vi "Tester.vi"() -> ()   [LabVIEW 2019, in "BigMAQ.lvclass"]
uses:
  BigMAQ.lvclass
  <userlib>/Levylab/Relay Box/Typedefs/Resistor--enum.ctl
  BigMAQ.lvclass/BigMAQ.ctl
  <userlib>/Levylab/Relay Box/Relay-Box.lvclass
panel:
  out "Array":i32[](array[numeric])
  out "x = y?":bool
  out "Image":T1(plugin-control)
  in  "Collapse":bool
  out "Render":T1(plugin-control)
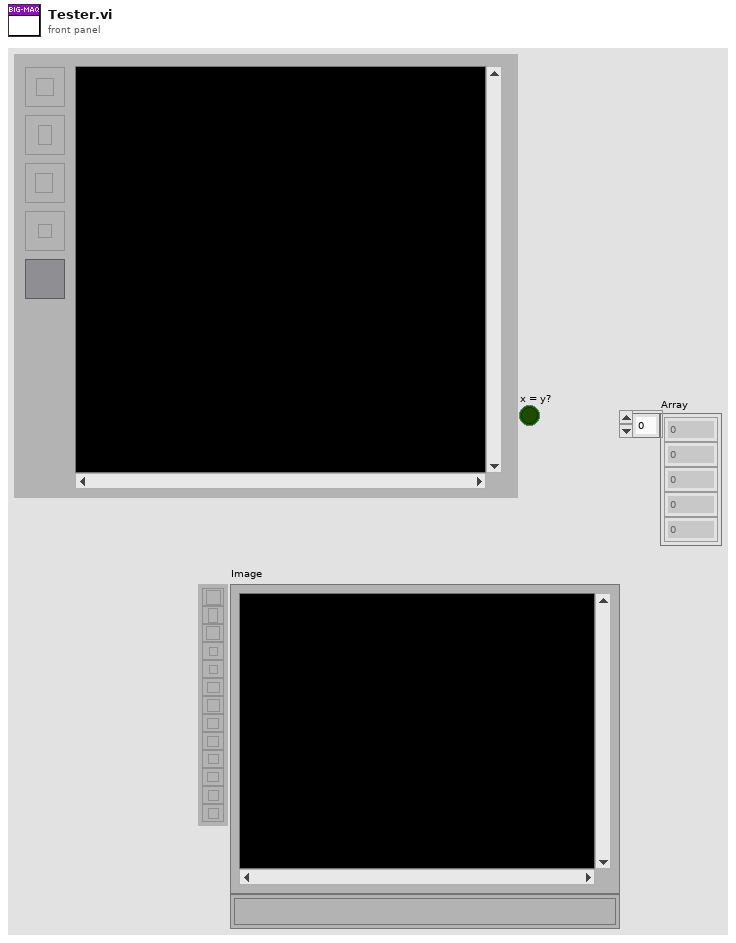
[diagram p1: front panel]
types:
  T1 = typedef "IMAQ Image.ctl" = refnum<image>
  T2 = typedef "Relay-Box.lvclass/Resistor--enum.ctl" = enum16{"open", "discharge tip", "0 ohms", "100k ohm", "10M ohm", "1G ohm"}
  T3 = cluster{"Name":string, "Litho":cluster{"X":dbl, "Y":dbl, "Speed":dbl, "Voltage":dbl}[], "Set Resistance":T2, "Meta":variant}[]
  T4 = cluster{"Name":string, "Litho":cluster{"X":dbl, "Y":dbl, "Speed":dbl, "Voltage":dbl}[], "Set Resistance":T2, "Meta":variant}
  T5 = cluster{"X":dbl, "Y":dbl, "Speed":dbl, "Voltage":dbl}[]
  T6 = cluster{"X":dbl, "Y":dbl, "Speed":dbl, "Voltage":dbl}
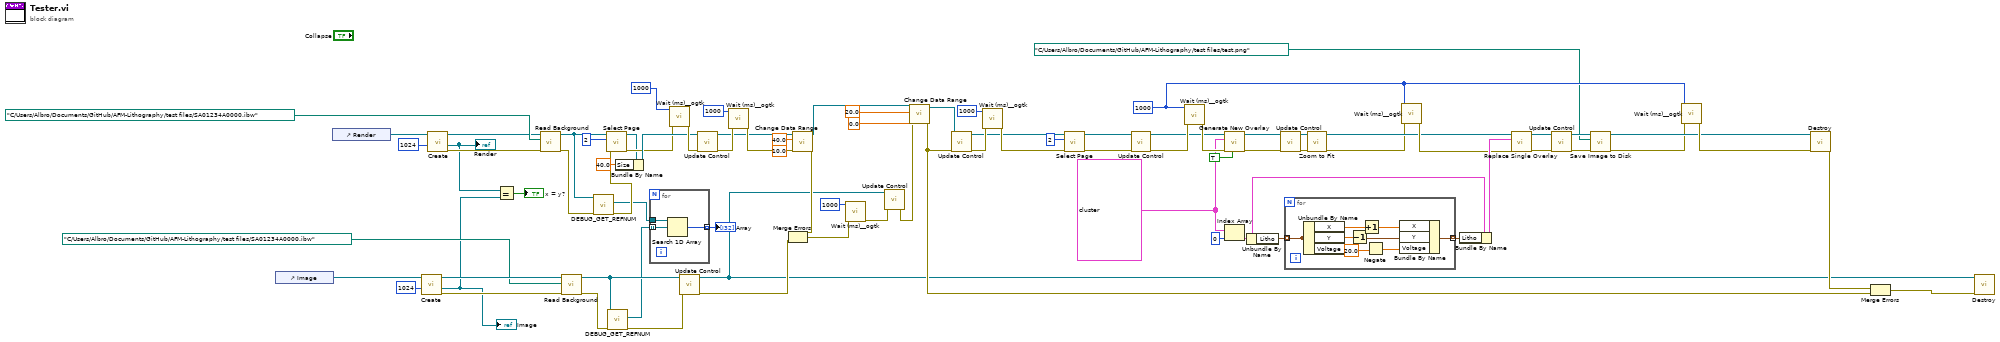
[diagram p0: block diagram]
diagram:
  w63 = T3 [{"Name"="p0", "Litho"=array[26726 elements], "Set Resistance"=enum."1G ohm", "Meta"=variant}, {"Name"="p1", "Litho"=array[12429 elements], "Set Resistance"=enum."1G ohm", "Meta"=variant}, {"Name"="p2", "Litho"=array[8953 elements], "Set Resistance"=enum."1G ohm", "Meta"=variant}, {"Name"="p3", "Litho"=array[11526 elements], "Set Resistance"=enum."1G ohm", "Meta"=variant}, {"Name"="p4", "Litho"=array[11508 elements], "Set Resistance"=enum."1G ohm", "Meta"=variant}, {"Name"="p5", "Litho"=array[11203 elements], "Set Resistance"=enum."1G ohm", "Meta"=variant}, {"Name"="p6", "Litho"=array[9937 elements], "Set Resistance"=enum."1G ohm", "Meta"=variant}, {"Name"="p7", "Litho"=array[9921 elements], "Set Resistance"=enum."1G ohm", "Meta"=variant}, {"Name"="p8", "Litho"=array[9914 elements], "Set Resistance"=enum."1G ohm", "Meta"=variant}, {"Name"="p9", "Litho"=array[57227 elements], "Set Resistance"=enum."1G ohm", "Meta"=variant}, {"Name"="f0", "Litho"=[{"X"=5.710942899999999, "Y"=17.975706, "Speed"=10.0, "Voltage"=10.0}, {"X"=6.38914543287037, "Y"=17.336981402777777, "Speed"=10.0, "Voltage"=10.0}, {"X"=7.122646896296295, "Y"=16.828463888888884, "Speed"=10.0, "Voltage"=10.0}, {"X"=7.9028574875, "Y"=16.429927874999997, "Speed"=10.0, "Voltage"=10.0}, {"X"=8.721187403703704, "Y"=16.121147777777775, "Speed"=10.0, "Voltage"=10.0}, {"X"=9.56904684212963, "Y"=15.88189801388889, "Speed"=10.0, "Voltage"=10.0}, {"X"=10.437846, "Y"=15.691952999999998, "Speed"=10.0, "Voltage"=10.0}, {"X"=9.579383034722223, "Y"=15.781785605555555, "Speed"=10.0, "Voltage"=10.0}, {"X"=8.740301544444446, "Y"=15.905736977777776, "Speed"=10.0, "Voltage"=10.0}, {"X"=7.9277050875, "Y"=16.079518349999997, "Speed"=10.0, "Voltage"=10.0}, {"X"=7.148697222222221, "Y"=16.31884095555555, "Speed"=10.0, "Voltage"=10.0}, {"X"=6.410381506944445, "Y"=16.639416027777777, "Speed"=10.0, "Voltage"=10.0}, {"X"=5.719861499999999, "Y"=17.056954799999996, "Speed"=10.0, "Voltage"=10.0}, {"X"=5.728780099999999, "Y"=16.138203599999997, "Speed"=10.0, "Voltage"=10.0}, {"X"=6.431617581018519, "Y"=15.941850652777777, "Speed"=10.0, "Voltage"=10.0}, {"X"=7.174747548148147, "Y"=15.809218022222218, "Speed"=10.0, "Voltage"=10.0}, {"X"=7.952552687499999, "Y"=15.729108824999997, "Speed"=10.0, "Voltage"=10.0}, {"X"=8.759415685185186, "Y"=15.690326177777777, "Speed"=10.0, "Voltage"=10.0}, {"X"=9.589719227314816, "Y"=15.68167319722222, "Speed"=10.0, "Voltage"=10.0}, {"X"=10.437846, "Y"=15.691952999999998, "Speed"=10.0, "Voltage"=10.0}, {"X"=9.60005541990741, "Y"=15.581560788888888, "Speed"=10.0, "Voltage"=10.0}, {"X"=8.778529825925926, "Y"=15.474915377777776, "Speed"=10.0, "Voltage"=10.0}, {"X"=7.9774002875, "Y"=15.378699299999997, "Speed"=10.0, "Voltage"=10.0}, {"X"=7.200797874074075, "Y"=15.299595088888886, "Speed"=10.0, "Voltage"=10.0}, {"X"=6.452853655092593, "Y"=15.244285277777777, "Speed"=10.0, "Voltage"=10.0}, {"X"=5.737698699999999, "Y"=15.219452399999996, "Speed"=10.0, "Voltage"=10.0}, {"X"=5.7466173, "Y"=14.300701199999995, "Speed"=10.0, "Voltage"=10.0}, {"X"=6.474089729166667, "Y"=14.546719902777777, "Speed"=10.0, "Voltage"=10.0}, {"X"=7.226848200000001, "Y"=14.789972155555553, "Speed"=10.0, "Voltage"=10.0}, {"X"=8.0022478875, "Y"=15.028289774999998, "Speed"=10.0, "Voltage"=10.0}, {"X"=8.797643966666667, "Y"=15.259504577777776, "Speed"=10.0, "Voltage"=10.0}, {"X"=9.610391612500003, "Y"=15.481448380555555, "Speed"=10.0, "Voltage"=10.0}, {"X"=10.437846, "Y"=15.691952999999998, "Speed"=10.0, "Voltage"=10.0}, {"X"=9.620727805092596, "Y"=15.381335972222221, "Speed"=10.0, "Voltage"=10.0}, {"X"=8.816758107407408, "Y"=15.044093777777777, "Speed"=10.0, "Voltage"=10.0}, {"X"=8.027095487499999, "Y"=14.677880249999998, "Speed"=10.0, "Voltage"=10.0}, {"X"=7.252898525925927, "Y"=14.280349222222222, "Speed"=10.0, "Voltage"=10.0}, {"X"=6.495325803240741, "Y"=13.849154527777776, "Speed"=10.0, "Voltage"=10.0}, {"X"=5.7555359, "Y"=13.381949999999996, "Speed"=10.0, "Voltage"=10.0}], "Set Resistance"=enum."open", "Meta"=variant}, {"Name"="f1", "Litho"=[{"X"=13.400891999999999, "Y"=10.059383, "Speed"=10.0, "Voltage"=10.0}, {"X"=14.039616597222224, "Y"=10.737586125, "Speed"=10.0, "Voltage"=10.0}, {"X"=14.548134111111112, "Y"=11.471087999999998, "Speed"=10.0, "Voltage"=10.0}, {"X"=14.946670125, "Y"=12.251298874999998, "Speed"=10.0, "Voltage"=10.0}, {"X"=15.255450222222224, "Y"=13.069628999999999, "Speed"=10.0, "Voltage"=10.0}, {"X"=15.494699986111113, "Y"=13.917488625, "Speed"=10.0, "Voltage"=10.0}, {"X"=15.684645, "Y"=14.786287999999999, "Speed"=10.0, "Voltage"=10.0}, {"X"=15.594812394444446, "Y"=13.92782480462963, "Speed"=10.0, "Voltage"=10.0}, {"X"=15.470861022222223, "Y"=13.088743103703703, "Speed"=10.0, "Voltage"=10.0}, {"X"=15.29707965, "Y"=12.276146424999999, "Speed"=10.0, "Voltage"=10.0}, {"X"=15.057757044444447, "Y"=11.497138296296296, "Speed"=10.0, "Voltage"=10.0}, {"X"=14.737181972222224, "Y"=10.758822245370371, "Speed"=10.0, "Voltage"=10.0}, {"X"=14.3196432, "Y"=10.0683018, "Speed"=10.0, "Voltage"=10.0}, {"X"=15.2383944, "Y"=10.0772206, "Speed"=10.0, "Voltage"=10.0}, {"X"=15.434747347222224, "Y"=10.780058365740741, "Speed"=10.0, "Voltage"=10.0}, {"X"=15.56737997777778, "Y"=11.523188592592591, "Speed"=10.0, "Voltage"=10.0}, {"X"=15.647489175, "Y"=12.300993975, "Speed"=10.0, "Voltage"=10.0}, {"X"=15.686271822222224, "Y"=13.107857207407406, "Speed"=10.0, "Voltage"=10.0}, {"X"=15.69492480277778, "Y"=13.938160984259259, "Speed"=10.0, "Voltage"=10.0}, {"X"=15.684645, "Y"=14.786287999999999, "Speed"=10.0, "Voltage"=10.0}, {"X"=15.795037211111115, "Y"=13.94849716388889, "Speed"=10.0, "Voltage"=10.0}, {"X"=15.901682622222225, "Y"=13.12697131111111, "Speed"=10.0, "Voltage"=10.0}, {"X"=15.9978987, "Y"=12.325841525000001, "Speed"=10.0, "Voltage"=10.0}, {"X"=16.077002911111112, "Y"=11.549238888888887, "Speed"=10.0, "Voltage"=10.0}, {"X"=16.132312722222224, "Y"=10.80129448611111, "Speed"=10.0, "Voltage"=10.0}, {"X"=16.1571456, "Y"=10.0861394, "Speed"=10.0, "Voltage"=10.0}, {"X"=17.075896800000002, "Y"=10.0950582, "Speed"=10.0, "Voltage"=10.0}, {"X"=16.829878097222224, "Y"=10.82253060648148, "Speed"=10.0, "Voltage"=10.0}, {"X"=16.586625844444445, "Y"=11.575289185185184, "Speed"=10.0, "Voltage"=10.0}, {"X"=16.348308225, "Y"=12.350689075, "Speed"=10.0, "Voltage"=10.0}, {"X"=16.117093422222226, "Y"=13.146085414814813, "Speed"=10.0, "Voltage"=10.0}, {"X"=15.895149619444448, "Y"=13.958833343518519, "Speed"=10.0, "Voltage"=10.0}, {"X"=15.684645, "Y"=14.786287999999999, "Speed"=10.0, "Voltage"=10.0}, {"X"=15.99526202777778, "Y"=13.969169523148148, "Speed"=10.0, "Voltage"=10.0}, {"X"=16.332504222222223, "Y"=13.165199518518516, "Speed"=10.0, "Voltage"=10.0}, {"X"=16.69871775, "Y"=12.375536625, "Speed"=10.0, "Voltage"=10.0}, {"X"=17.096248777777777, "Y"=11.601339481481482, "Speed"=10.0, "Voltage"=10.0}, {"X"=17.527443472222224, "Y"=10.84376672685185, "Speed"=10.0, "Voltage"=10.0}, {"X"=17.994648, "Y"=10.103976999999999, "Speed"=10.0, "Voltage"=10.0}], "Set Resistance"=enum."open", "Meta"=variant}, {"Name"="f2", "Litho"=[{"X"=18.739549, "Y"=9.9886728, "Speed"=10.0, "Voltage"=10.0}, {"X"=19.378273597222226, "Y"=10.666875587962963, "Speed"=10.0, "Voltage"=10.0}, {"X"=19.88679111111111, "Y"=11.400377237037036, "Speed"=10.0, "Voltage"=10.0}, {"X"=20.285327125000002, "Y"=12.180587974999998, "Speed"=10.0, "Voltage"=10.0}, {"X"=20.59410722222222, "Y"=12.998918029629628, "Speed"=10.0, "Voltage"=10.0}, {"X"=20.833356986111113, "Y"=13.846777628703705, "Speed"=10.0, "Voltage"=10.0}, {"X"=21.023302, "Y"=14.715577, "Speed"=10.0, "Voltage"=10.0}, {"X"=20.933469394444444, "Y"=13.857113821481484, "Speed"=10.0, "Voltage"=10.0}, {"X"=20.80951802222222, "Y"=13.018032171851852, "Speed"=10.0, "Voltage"=10.0}, {"X"=20.63573665, "Y"=12.20543558, "Speed"=10.0, "Voltage"=10.0}, {"X"=20.39641404444444, "Y"=11.426427574814815, "Speed"=10.0, "Voltage"=10.0}, {"X"=20.07583897222223, "Y"=10.688111685185184, "Speed"=10.0, "Voltage"=10.0}, {"X"=19.6583002, "Y"=9.99759144, "Speed"=10.0, "Voltage"=10.0}, {"X"=20.5770514, "Y"=10.00651008, "Speed"=10.0, "Voltage"=10.0}, {"X"=20.77340434722223, "Y"=10.709347782407407, "Speed"=10.0, "Voltage"=10.0}, {"X"=20.906036977777777, "Y"=11.452477912592592, "Speed"=10.0, "Voltage"=10.0}, {"X"=20.986146175, "Y"=12.230283184999998, "Speed"=10.0, "Voltage"=10.0}, {"X"=21.024928822222222, "Y"=13.037146314074073, "Speed"=10.0, "Voltage"=10.0}, {"X"=21.03358180277778, "Y"=13.867450014259262, "Speed"=10.0, "Voltage"=10.0}, {"X"=21.023302, "Y"=14.715577, "Speed"=10.0, "Voltage"=10.0}, {"X"=21.133694211111113, "Y"=13.877786207037037, "Speed"=10.0, "Voltage"=10.0}, {"X"=21.240339622222223, "Y"=13.056260456296295, "Speed"=10.0, "Voltage"=10.0}, {"X"=21.336555699999998, "Y"=12.255130789999999, "Speed"=10.0, "Voltage"=10.0}, {"X"=21.415659911111113, "Y"=11.47852825037037, "Speed"=10.0, "Voltage"=10.0}, {"X"=21.47096972222223, "Y"=10.73058387962963, "Speed"=10.0, "Voltage"=10.0}, {"X"=21.495802599999998, "Y"=10.01542872, "Speed"=10.0, "Voltage"=10.0}, {"X"=22.414553799999997, "Y"=10.024347359999998, "Speed"=10.0, "Voltage"=10.0}, {"X"=22.16853509722223, "Y"=10.751819976851852, "Speed"=10.0, "Voltage"=10.0}, {"X"=21.925282844444446, "Y"=11.50457858814815, "Speed"=10.0, "Voltage"=10.0}, {"X"=21.686965224999998, "Y"=12.279978394999997, "Speed"=10.0, "Voltage"=10.0}, {"X"=21.455750422222224, "Y"=13.075374598518518, "Speed"=10.0, "Voltage"=10.0}, {"X"=21.233806619444444, "Y"=13.888122399814815, "Speed"=10.0, "Voltage"=10.0}, {"X"=21.023302, "Y"=14.715577, "Speed"=10.0, "Voltage"=10.0}, {"X"=21.333919027777778, "Y"=13.898458592592593, "Speed"=10.0, "Voltage"=10.0}, {"X"=21.671161222222224, "Y"=13.09448874074074, "Speed"=10.0, "Voltage"=10.0}, {"X"=22.037374749999998, "Y"=12.304825999999998, "Speed"=10.0, "Voltage"=10.0}, {"X"=22.43490577777778, "Y"=11.530628925925928, "Speed"=10.0, "Voltage"=10.0}, {"X"=22.86610047222223, "Y"=10.773056074074074, "Speed"=10.0, "Voltage"=10.0}, {"X"=23.333305, "Y"=10.033266, "Speed"=10.0, "Voltage"=10.0}], "Set Resistance"=enum."open", "Meta"=variant}, {"Name"="f3", "Litho"=[{"X"=8.1004383, "Y"=10.879120000000002, "Speed"=10.0, "Voltage"=10.0}, {"X"=8.862424111111112, "Y"=11.415129314814816, "Speed"=10.0, "Voltage"=10.0}, {"X"=9.507971822222222, "Y"=12.031475851851853, "Speed"=10.0, "Voltage"=10.0}, {"X"=10.055168250000001, "Y"=12.715680500000001, "Speed"=10.0, "Voltage"=10.0}, {"X"=10.522100211111113, "Y"=13.455264148148153, "Speed"=10.0, "Voltage"=10.0}, {"X"=10.926854522222225, "Y"=14.23774768518519, "Speed"=10.0, "Voltage"=10.0}, {"X"=11.287518, "Y"=15.050652000000003, "Speed"=10.0, "Voltage"=10.0}, {"X"=11.027001790925928, "Y"=14.227754495833338, "Speed"=10.0, "Voltage"=10.0}, {"X"=10.736957754074075, "Y"=13.430699566666672, "Speed"=10.0, "Voltage"=10.0}, {"X"=10.403422675000002, "Y"=12.669603187500002, "Speed"=10.0, "Voltage"=10.0}, {"X"=10.012433339259259, "Y"=11.954581333333335, "Speed"=10.0, "Voltage"=10.0}, {"X"=9.550026532407408, "Y"=11.295749979166668, "Speed"=10.0, "Voltage"=10.0}, {"X"=9.00223904, "Y"=10.703225100000001, "Speed"=10.0, "Voltage"=10.0}, {"X"=9.90403978, "Y"=10.527330200000002, "Speed"=10.0, "Voltage"=10.0}, {"X"=10.237628953703705, "Y"=11.176370643518519, "Speed"=10.0, "Voltage"=10.0}, {"X"=10.516894856296297, "Y"=11.877686814814817, "Speed"=10.0, "Voltage"=10.0}, {"X"=10.751677100000002, "Y"=12.623525875000002, "Speed"=10.0, "Voltage"=10.0}, {"X"=10.951815297037037, "Y"=13.40613498518519, "Speed"=10.0, "Voltage"=10.0}, {"X"=11.12714905962963, "Y"=14.217761306481485, "Speed"=10.0, "Voltage"=10.0}, {"X"=11.287518000000002, "Y"=15.050652000000001, "Speed"=10.0, "Voltage"=10.0}, {"X"=11.227296328333335, "Y"=14.207768117129632, "Speed"=10.0, "Voltage"=10.0}, {"X"=11.166672839999999, "Y"=13.381570403703705, "Speed"=10.0, "Voltage"=10.0}, {"X"=11.099931524999999, "Y"=12.577448562500003, "Speed"=10.0, "Voltage"=10.0}, {"X"=11.021356373333333, "Y"=11.800792296296297, "Speed"=10.0, "Voltage"=10.0}, {"X"=10.925231375, "Y"=11.056991307870371, "Speed"=10.0, "Voltage"=10.0}, {"X"=10.80584052, "Y"=10.3514353, "Speed"=10.0, "Voltage"=10.0}, {"X"=11.707641259999999, "Y"=10.1755404, "Speed"=10.0, "Voltage"=10.0}, {"X"=11.612833796296297, "Y"=10.937611972222223, "Speed"=10.0, "Voltage"=10.0}, {"X"=11.52581789037037, "Y"=11.723897777777779, "Speed"=10.0, "Voltage"=10.0}, {"X"=11.44818595, "Y"=12.531371250000001, "Speed"=10.0, "Voltage"=10.0}, {"X"=11.38153038296296, "Y"=13.357005822222224, "Speed"=10.0, "Voltage"=10.0}, {"X"=11.327443597037039, "Y"=14.19777492777778, "Speed"=10.0, "Voltage"=10.0}, {"X"=11.287518, "Y"=15.050652000000003, "Speed"=10.0, "Voltage"=10.0}, {"X"=11.287518, "Y"=15.050652000000001, "Speed"=10.0, "Voltage"=10.0}, {"X"=11.427590865740742, "Y"=14.187781738425928, "Speed"=10.0, "Voltage"=10.0}, {"X"=11.596387925925924, "Y"=13.33244124074074, "Speed"=10.0, "Voltage"=10.0}, {"X"=11.796440375, "Y"=12.485293937500002, "Speed"=10.0, "Voltage"=10.0}, {"X"=12.030279407407408, "Y"=11.647003259259261, "Speed"=10.0, "Voltage"=10.0}, {"X"=12.300436217592592, "Y"=10.818232636574074, "Speed"=10.0, "Voltage"=10.0}, {"X"=12.609442, "Y"=9.9996455, "Speed"=10.0, "Voltage"=10.0}], "Set Resistance"=enum."open", "Meta"=variant}, {"Name"="f4", "Litho"=[{"X"=28.994557, "Y"=10.486845999999998, "Speed"=10.0, "Voltage"=10.0}, {"X"=28.186134203703702, "Y"=10.958520509259259, "Speed"=10.0, "Voltage"=10.0}, {"X"=27.47246962962963, "Y"=11.504807740740741, "Speed"=10.0, "Voltage"=10.0}, {"X"=26.84426, "Y"=12.118856749999999, "Speed"=10.0, "Voltage"=10.0}, {"X"=26.292202037037036, "Y"=12.793816592592592, "Speed"=10.0, "Voltage"=10.0}, {"X"=25.806992462962963, "Y"=13.522836324074074, "Speed"=10.0, "Voltage"=10.0}, {"X"=25.379327999999997, "Y"=14.299064999999999, "Speed"=10.0, "Voltage"=10.0}, {"X"=25.715396165740742, "Y"=13.50474573064815, "Speed"=10.0, "Voltage"=10.0}, {"X"=26.106198525925926, "Y"=12.75046851185185, "Speed"=10.0, "Voltage"=10.0}, {"X"=26.551395874999997, "Y"=12.0412214275, "Speed"=10.0, "Voltage"=10.0}, {"X"=27.050649007407408, "Y"=11.381992561481482, "Speed"=10.0, "Voltage"=10.0}, {"X"=27.60361871759259, "Y"=10.777769997685187, "Speed"=10.0, "Voltage"=10.0}, {"X"=28.2099658, "Y"=10.23354182, "Speed"=10.0, "Voltage"=10.0}, {"X"=27.425374599999998, "Y"=9.980237639999999, "Speed"=10.0, "Voltage"=10.0}, {"X"=27.02110323148148, "Y"=10.597019486111112, "Speed"=10.0, "Voltage"=10.0}, {"X"=26.628828385185184, "Y"=11.259177382222223, "Speed"=10.0, "Voltage"=10.0}, {"X"=26.258531749999996, "Y"=11.963586105000001, "Speed"=10.0, "Voltage"=10.0}, {"X"=25.920195014814816, "Y"=12.707120431111111, "Speed"=10.0, "Voltage"=10.0}, {"X"=25.623799868518518, "Y"=13.486655137222224, "Speed"=10.0, "Voltage"=10.0}, {"X"=25.379327999999994, "Y"=14.299065, "Speed"=10.0, "Voltage"=10.0}, {"X"=25.532203571296293, "Y"=13.468564543796298, "Speed"=10.0, "Voltage"=10.0}, {"X"=25.734191503703705, "Y"=12.663772350370369, "Speed"=10.0, "Voltage"=10.0}, {"X"=25.965667625000002, "Y"=11.8859507825, "Speed"=10.0, "Voltage"=10.0}, {"X"=26.207007762962963, "Y"=11.136362202962964, "Speed"=10.0, "Voltage"=10.0}, {"X"=26.43858774537037, "Y"=10.41626897453704, "Speed"=10.0, "Voltage"=10.0}, {"X"=26.640783399999997, "Y"=9.726933459999998, "Speed"=10.0, "Voltage"=10.0}, {"X"=25.856192199999995, "Y"=9.473629279999999, "Speed"=10.0, "Voltage"=10.0}, {"X"=25.85607225925926, "Y"=10.235518462962965, "Speed"=10.0, "Voltage"=10.0}, {"X"=25.785187140740742, "Y"=11.013547023703705, "Speed"=10.0, "Voltage"=10.0}, {"X"=25.6728035, "Y"=11.80831546, "Speed"=10.0, "Voltage"=10.0}, {"X"=25.548187992592595, "Y"=12.62042426962963, "Speed"=10.0, "Voltage"=10.0}, {"X"=25.440607274074072, "Y"=13.450473950370371, "Speed"=10.0, "Voltage"=10.0}, {"X"=25.379327999999997, "Y"=14.299064999999999, "Speed"=10.0, "Voltage"=10.0}, {"X"=25.34901097685185, "Y"=13.432383356944445, "Speed"=10.0, "Voltage"=10.0}, {"X"=25.36218448148148, "Y"=12.577076188888888, "Speed"=10.0, "Voltage"=10.0}, {"X"=25.379939375, "Y"=11.7306801375, "Speed"=10.0, "Voltage"=10.0}, {"X"=25.363366518518518, "Y"=10.890731844444446, "Speed"=10.0, "Voltage"=10.0}, {"X"=25.27355677314815, "Y"=10.054767951388891, "Speed"=10.0, "Voltage"=10.0}, {"X"=25.071600999999998, "Y"=9.2203251, "Speed"=10.0, "Voltage"=10.0}], "Set Resistance"=enum."open", "Meta"=variant}, {"Name"="f5", "Litho"=[{"X"=31.708383, "Y"=17.654207, "Speed"=10.0, "Voltage"=10.0}, {"X"=31.030180717592593, "Y"=17.015482402777778, "Speed"=10.0, "Voltage"=10.0}, {"X"=30.296679407407403, "Y"=16.506964888888888, "Speed"=10.0, "Voltage"=10.0}, {"X"=29.516468875, "Y"=16.108428875, "Speed"=10.0, "Voltage"=10.0}, {"X"=28.69813892592593, "Y"=15.799648777777778, "Speed"=10.0, "Voltage"=10.0}, {"X"=27.850279365740747, "Y"=15.560399013888887, "Speed"=10.0, "Voltage"=10.0}, {"X"=26.98148, "Y"=15.370453999999999, "Speed"=10.0, "Voltage"=10.0}, {"X"=27.839943173148153, "Y"=15.460286605555552, "Speed"=10.0, "Voltage"=10.0}, {"X"=28.67902478518519, "Y"=15.584237977777777, "Speed"=10.0, "Voltage"=10.0}, {"X"=29.491621275, "Y"=15.75801935, "Speed"=10.0, "Voltage"=10.0}, {"X"=30.27062908148148, "Y"=15.997341955555555, "Speed"=10.0, "Voltage"=10.0}, {"X"=31.00894464351852, "Y"=16.317917027777778, "Speed"=10.0, "Voltage"=10.0}, {"X"=31.699464400000004, "Y"=16.7354558, "Speed"=10.0, "Voltage"=10.0}, {"X"=31.690545800000002, "Y"=15.816704599999998, "Speed"=10.0, "Voltage"=10.0}, {"X"=30.98770856944445, "Y"=15.620351652777776, "Speed"=10.0, "Voltage"=10.0}, {"X"=30.24457875555556, "Y"=15.487719022222223, "Speed"=10.0, "Voltage"=10.0}, {"X"=29.466773675, "Y"=15.407609824999998, "Speed"=10.0, "Voltage"=10.0}, {"X"=28.65991064444445, "Y"=15.368827177777776, "Speed"=10.0, "Voltage"=10.0}, {"X"=27.82960698055556, "Y"=15.36017419722222, "Speed"=10.0, "Voltage"=10.0}, {"X"=26.981480000000005, "Y"=15.370453999999997, "Speed"=10.0, "Voltage"=10.0}, {"X"=27.819270787962967, "Y"=15.260061788888889, "Speed"=10.0, "Voltage"=10.0}, {"X"=28.640796503703708, "Y"=15.153416377777777, "Speed"=10.0, "Voltage"=10.0}, {"X"=29.441926074999998, "Y"=15.057200299999998, "Speed"=10.0, "Voltage"=10.0}, {"X"=30.218528429629632, "Y"=14.978096088888888, "Speed"=10.0, "Voltage"=10.0}, {"X"=30.966472495370372, "Y"=14.922786277777778, "Speed"=10.0, "Voltage"=10.0}, {"X"=31.6816272, "Y"=14.897953399999999, "Speed"=10.0, "Voltage"=10.0}, {"X"=31.6727086, "Y"=13.979202199999998, "Speed"=10.0, "Voltage"=10.0}, {"X"=30.9452364212963, "Y"=14.225220902777776, "Speed"=10.0, "Voltage"=10.0}, {"X"=30.19247810370371, "Y"=14.468473155555554, "Speed"=10.0, "Voltage"=10.0}, {"X"=29.417078474999997, "Y"=14.706790774999998, "Speed"=10.0, "Voltage"=10.0}, {"X"=28.621682362962964, "Y"=14.938005577777776, "Speed"=10.0, "Voltage"=10.0}, {"X"=27.808934595370374, "Y"=15.159949380555556, "Speed"=10.0, "Voltage"=10.0}, {"X"=26.98148, "Y"=15.370453999999999, "Speed"=10.0, "Voltage"=10.0}, {"X"=27.79859840277778, "Y"=15.059836972222222, "Speed"=10.0, "Voltage"=10.0}, {"X"=28.602568222222224, "Y"=14.722594777777775, "Speed"=10.0, "Voltage"=10.0}, {"X"=29.392230875, "Y"=14.356381249999997, "Speed"=10.0, "Voltage"=10.0}, {"X"=30.166427777777788, "Y"=13.958850222222221, "Speed"=10.0, "Voltage"=10.0}, {"X"=30.924000347222226, "Y"=13.527655527777775, "Speed"=10.0, "Voltage"=10.0}, {"X"=31.663790000000002, "Y"=13.060450999999997, "Speed"=10.0, "Voltage"=10.0}], "Set Resistance"=enum."open", "Meta"=variant}, {"Name"="r0", "Litho"=[{"X"=14.347161, "Y"=28.2297925, "Speed"=10.0, "Voltage"=10.0}, {"X"=26.235564, "Y"=28.2297925, "Speed"=10.0, "Voltage"=10.0}, {"X"=14.347161, "Y"=27.3228159375, "Speed"=10.0, "Voltage"=10.0}, {"X"=26.235564, "Y"=27.3228159375, "Speed"=10.0, "Voltage"=10.0}, {"X"=14.347161, "Y"=26.415839374999997, "Speed"=10.0, "Voltage"=10.0}, {"X"=26.235564, "Y"=26.415839374999997, "Speed"=10.0, "Voltage"=10.0}, {"X"=14.347161, "Y"=25.5088628125, "Speed"=10.0, "Voltage"=10.0}, {"X"=26.235564, "Y"=25.5088628125, "Speed"=10.0, "Voltage"=10.0}, {"X"=14.347161, "Y"=24.60188625, "Speed"=10.0, "Voltage"=10.0}, {"X"=26.235564, "Y"=24.60188625, "Speed"=10.0, "Voltage"=10.0}, {"X"=14.347161, "Y"=23.6949096875, "Speed"=10.0, "Voltage"=10.0}, {"X"=26.235564, "Y"=23.6949096875, "Speed"=10.0, "Voltage"=10.0}, {"X"=14.347161, "Y"=22.787933125000002, "Speed"=10.0, "Voltage"=10.0}, {"X"=26.235564, "Y"=22.787933125000002, "Speed"=10.0, "Voltage"=10.0}, {"X"=14.347161, "Y"=21.8809565625, "Speed"=10.0, "Voltage"=10.0}, {"X"=26.235564, "Y"=21.8809565625, "Speed"=10.0, "Voltage"=10.0}], "Set Resistance"=enum."open", "Meta"=variant}, {"Name"="r1", "Litho"=[{"X"=5.548541376041481, "Y"=37.48831096835694, "Speed"=10.0, "Voltage"=10.0}, {"X"=17.11359627236498, "Y"=37.45427714309987, "Speed"=10.0, "Voltage"=10.0}, {"X"=5.2166337533397185, "Y"=36.57868963636656, "Speed"=10.0, "Voltage"=10.0}, {"X"=16.781688649663216, "Y"=36.54465581110949, "Speed"=10.0, "Voltage"=10.0}, {"X"=4.884726130637957, "Y"=35.66906830437618, "Speed"=10.0, "Voltage"=10.0}, {"X"=16.449781026961457, "Y"=35.63503447911911, "Speed"=10.0, "Voltage"=10.0}, {"X"=4.552818507936195, "Y"=34.7594469723858, "Speed"=10.0, "Voltage"=10.0}, {"X"=16.117873404259694, "Y"=34.725413147128734, "Speed"=10.0, "Voltage"=10.0}, {"X"=4.220910885234433, "Y"=33.84982564039542, "Speed"=10.0, "Voltage"=10.0}, {"X"=15.785965781557934, "Y"=33.81579181513835, "Speed"=10.0, "Voltage"=10.0}, {"X"=3.889003262532671, "Y"=32.94020430840504, "Speed"=10.0, "Voltage"=10.0}, {"X"=15.45405815885617, "Y"=32.90617048314797, "Speed"=10.0, "Voltage"=10.0}, {"X"=3.5570956398309095, "Y"=32.030582976414664, "Speed"=10.0, "Voltage"=10.0}, {"X"=15.12215053615441, "Y"=31.996549151157588, "Speed"=10.0, "Voltage"=10.0}, {"X"=3.225188017129147, "Y"=31.120961644424288, "Speed"=10.0, "Voltage"=10.0}, {"X"=14.790242913452648, "Y"=31.086927819167208, "Speed"=10.0, "Voltage"=10.0}, {"X"=2.8932803944273853, "Y"=30.211340312433908, "Speed"=10.0, "Voltage"=10.0}, {"X"=14.458335290750886, "Y"=30.17730648717683, "Speed"=10.0, "Voltage"=10.0}, {"X"=2.561372771725623, "Y"=29.30171898044353, "Speed"=10.0, "Voltage"=10.0}, {"X"=14.126427668049125, "Y"=29.267685155186445, "Speed"=10.0, "Voltage"=10.0}], "Set Resistance"=enum."open", "Meta"=variant}, {"Name"="d0", "Litho"=[], "Set Resistance"=enum."open", "Meta"=variant}, {"Name"="d1", "Litho"=[], "Set Resistance"=enum."open", "Meta"=variant}, {"Name"="d2", "Litho"=[], "Set Resistance"=enum."open", "Meta"=variant}, {"Name"="d3", "Litho"=[], "Set Resistance"=enum."open", "Meta"=variant}, {"Name"="d4", "Litho"=[], "Set Resistance"=enum."open", "Meta"=variant}, {"Name"="d5", "Litho"=[], "Set Resistance"=enum."open", "Meta"=variant}, {"Name"="d6", "Litho"=[], "Set Resistance"=enum."open", "Meta"=variant}, {"Name"="d7", "Litho"=[], "Set Resistance"=enum."open", "Meta"=variant}, {"Name"="d8", "Litho"=[], "Set Resistance"=enum."open", "Meta"=variant}] ("Lithography Data")
  w56 = u32 1000 ("milliseconds to wait")
  n1 = control-ref of="Image"() -> (w13:refnum<vi>)
  n2 = control-ref of="Render"() -> (w64:refnum<vi>)
  n3 = call "Create.vi"("Resolution"=1024, "Reference"=w13) -> ("error out"=w25:errorcluster, "To Control"=w11:T1, "BigMAQ out"=w26:refnum<class "BigMAQ.lvclass">)  [unwired: 7 in]
  "Image" <- w11
  n4 = call "Create.vi"("Resolution"=1024, "Reference"=w64) -> ("error out"=w80:errorcluster, "To Control"=w12:T1, "BigMAQ out"=w81:refnum<class "BigMAQ.lvclass">)  [unwired: 7 in]
  "Render" <- w12
  n5 = Equal?(x=w12, y=w11) -> (x = y?=→"x = y?":bool)
  n6 = call "Read Background.vi"("error in (no error)"=w80, "Path"=path "C:/Users/Albro/Documents/GitHub/AFM-Lithography/test files/SA01234A0000.ibw", "BigMAQ in"=w81) -> ("error out"=w5:errorcluster, "BigMAQ out"=w6:refnum<class "BigMAQ.lvclass">)  [unwired: 6 in, 1 out]
  n7 = call "Read Background.vi"("error in (no error)"=w25, "Path"=path "C:/Users/Albro/Documents/GitHub/AFM-Lithography/test files/SA01234A0000.ibw", "BigMAQ in"=w26) -> ("error out"=w8:errorcluster, "BigMAQ out"=w9:refnum<class "BigMAQ.lvclass">)  [unwired: 6 in, 1 out]
  n8 = call "DEBUG_GET_REFNUM.vi"("error in"=w5, "BigMAQ in"=w6) -> ("error out"=w4:errorcluster, "IMAQ REFNUMS"=w3:T1[])  [unwired: 7 in, 1 out]
  n9 = call "Select Page.vi"("error in (no error)"=w4, "Page"=2, "BigMAQ in"=w6) -> ("error out"=w33:errorcluster, "BigMAQ out"=w32:refnum<class "BigMAQ.lvclass">)  [unwired: 6 in, 1 out]
  n10 = call "DEBUG_GET_REFNUM.vi"("error in"=w8, "BigMAQ in"=w9) -> ("error out"=w7:errorcluster, "IMAQ REFNUMS"=w2:T1[])  [unwired: 7 in, 1 out]
  n11 = Bundle By Name(cluster=w32, "Size"=40.0) -> (w66:refnum<class "BigMAQ.lvclass">)
  n12 = for {
    tunnel: w3 -> [w85]
    tunnel: w2 -> [w84] mode=indexing
    tunnel: [w83] -> w1 mode=indexing
    n13 = Search 1D Array(1D array=w85, element=w84) -> (index of element=w83:i32)  [unwired: 1 in]
  }
  "Array" <- w1
  n14 = call <userlib>:"Wait (ms)__ogtk.vi"("error in (no error)"=w33, "milliseconds to wait"=u32 1000) -> ("error out"=w72:errorcluster)  [unwired: 8 in, 1 out]
  n15 = call "Update Control.vi"("error in"=w7, "BigMAQ in"=w9) -> ("error out"=w19:errorcluster, "BigMAQ out"=w14:refnum<class "BigMAQ.lvclass">)  [unwired: 8 in]
  n16 = call "Update Control.vi"("error in"=w72, "BigMAQ in"=w66) -> ("error out"=w77:errorcluster, "BigMAQ out"=w45:refnum<class "BigMAQ.lvclass">)  [unwired: 8 in]
  n17 = call <userlib>:"Wait (ms)__ogtk.vi"("error in (no error)"=w77, "milliseconds to wait"=u32 1000) -> ("error out"=w46:errorcluster)  [unwired: 8 in, 1 out]
  n18 = call "Change Data Range.vi"("error in"=w46, "Minimum"=sgl 10.0, "Maximum"=sgl 40.0, "BigMAQ in"=w45) -> ("error out"=w18:errorcluster, "BigMAQ out"=w29:refnum<class "BigMAQ.lvclass">)  [unwired: 6 in]
  n19 = Merge Errors(w18, w19) -> (w17:errorcluster)
  n20 = call <userlib>:"Wait (ms)__ogtk.vi"("error in (no error)"=w17, "milliseconds to wait"=u32 1000) -> ("error out"=w16:errorcluster)  [unwired: 8 in, 1 out]
  n21 = call "Update Control.vi"("error in"=w16, "BigMAQ in"=w14) -> ("error out"=w15:errorcluster)  [unwired: 8 in, 1 out]
  n22 = call "Change Data Range.vi"("error in"=w15, "Minimum"=sgl 0.0, "Maximum"=sgl 20.0, "BigMAQ in"=w29) -> ("error out"=w20:errorcluster, "BigMAQ out"=w28:refnum<class "BigMAQ.lvclass">)  [unwired: 6 in]
  n23 = call "Update Control.vi"("error in"=w20, "BigMAQ in"=w28) -> ("error out"=w49:errorcluster, "BigMAQ out"=w44:refnum<class "BigMAQ.lvclass">)  [unwired: 8 in]
  n24 = call <userlib>:"Wait (ms)__ogtk.vi"("error in (no error)"=w49, "milliseconds to wait"=u32 1000) -> ("error out"=w47:errorcluster)  [unwired: 8 in, 1 out]
  n25 = call "Select Page.vi"("error in (no error)"=w47, "Page"=2, "BigMAQ in"=w44) -> ("error out"=w75:errorcluster, "BigMAQ out"=w73:refnum<class "BigMAQ.lvclass">)  [unwired: 6 in, 1 out]
  n26 = call "Update Control.vi"("error in"=w75, "BigMAQ in"=w73) -> ("error out"=w74:errorcluster, "BigMAQ out"=w68:refnum<class "BigMAQ.lvclass">)  [unwired: 8 in]
  n27 = call <userlib>:"Wait (ms)__ogtk.vi"("error in (no error)"=w74, "milliseconds to wait"=w56) -> ("error out"=w71:errorcluster)  [unwired: 8 in, 1 out]
  n28 = call "Generate New Overlay.vi"("Label?"=TRUE, "error in"=w71, "Lithography Data"=w63, "BigMAQ in"=w68) -> ("error out"=w70:errorcluster, "BigMAQ out"=w69:refnum<class "BigMAQ.lvclass">)  [unwired: 6 in]
  n29 = Index Array(array=w63, index=0) -> (element=w59:T4)
  n30 = Unbundle By Name(w59) -> ("Litho"=w61:T5)
  n31 = call "Update Control.vi"("error in"=w70, "BigMAQ in"=w69) -> ("error out"=w52:errorcluster, "BigMAQ out"=w51:refnum<class "BigMAQ.lvclass">)  [unwired: 8 in]
  n32 = for {
    tunnel: w61 -> [w91] mode=indexing
    tunnel: [w87] -> w60 mode=indexing
    n33 = Unbundle By Name(w91) -> ("X"=w93:dbl, "Y"=w92:dbl)  [unwired: 1 out]
    n34 = Decrement(x=w92) -> (x-1=w89:dbl)
    n35 = Increment(x=w93) -> (x+1=w90:dbl)
    n36 = Negate(x=20.0) -> (-x=w88:dbl)
    n37 = Bundle By Name(cluster=w91, "X"=w90, "Y"=w89, "Voltage"=w88) -> (w87:T6)
  }
  n38 = call "Zoom to Fit.vi"("error in"=w52, "BigMAQ in"=w51) -> ("error out"=w40:errorcluster, "BigMAQ out"=w41:refnum<class "BigMAQ.lvclass">)  [unwired: 7 in, 1 out]
  n39 = call <userlib>:"Wait (ms)__ogtk.vi"("error in (no error)"=w40, "milliseconds to wait"=w56) -> ("error out"=w57:errorcluster)  [unwired: 8 in, 1 out]
  n40 = Bundle By Name(cluster=w59, "Litho"=w60) -> (w58:T4)
  n41 = call "Replace Single Overlay.vi"("error in"=w57, "Litho"=w58, "BigMAQ in"=w41) -> ("error out"=w54:errorcluster, "BigMAQ out"=w55:refnum<class "BigMAQ.lvclass">)  [unwired: 7 in]
  n42 = call "Update Control.vi"("error in"=w54, "BigMAQ in"=w55) -> ("error out"=w39:errorcluster, "BigMAQ out"=w36:refnum<class "BigMAQ.lvclass">)  [unwired: 8 in]
  n43 = call "Save Image to Disk.vi"("error in"=w39, "Path"=path "C:/Users/Albro/Documents/GitHub/AFM-Lithography/test files/test.png", "BigMAQ in"=w36) -> ("error out"=w37:errorcluster, "BigMAQ out"=w38:refnum<class "BigMAQ.lvclass">)  [unwired: 7 in]
  n44 = call <userlib>:"Wait (ms)__ogtk.vi"("error in (no error)"=w37, "milliseconds to wait"=w56) -> ("error out"=w53:errorcluster)  [unwired: 8 in, 1 out]
  n45 = call "Destroy.vi"("error in"=w53, "BigMAQ in"=w38) -> ("error out"=w22:errorcluster)  [unwired: 8 in, 1 out]
  n46 = Merge Errors(w22, w20) -> (w23:errorcluster)
  n47 = call "Destroy.vi"("error in"=w23, "BigMAQ in"=w14) -> ()  [unwired: 8 in, 2 out]
